vi "ClientNTTestInit.vi"(11 "Instance":u32) -> (3 "TestConfig":T1)   [LabVIEW 2019]
uses:
  ClientNTTestConfig.ctl
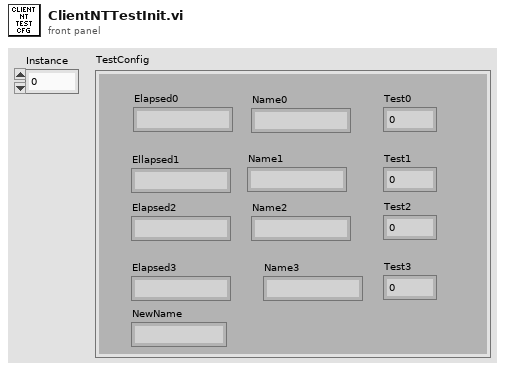
[diagram p1: front panel]
types:
  T1 = typedef "ClientNTTestConfig.ctl" = cluster{"Elapsed0":string, "Name0":string, "Test0":u32, "Ellapsed1":string, "Name1":string, "Test1":u32, "Elapsed2":string, "Name2":string, "Test2":u32, "Elapsed3":string, "Name3":string, "Test3":u32, "NewName":string}
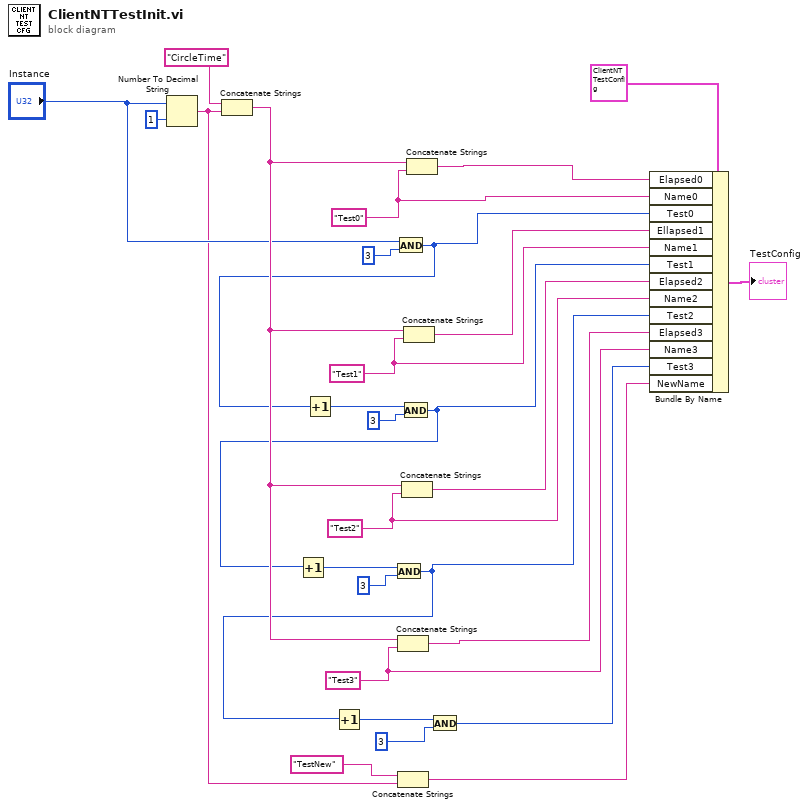
[diagram p0: block diagram]
diagram:
  w5 = "Test3" ("Name")
  w7 = "Test2" ("Name")
  w9 = "Test1" ("Name")
  w11 = "Test0" ("Name")
  n1 = Number To Decimal String(number="Instance", width (-)=i16 1) -> (decimal integer string=w3:string)
  n2 = Concatenate Strings("CircleTime" ("string"), w3) -> (w28:string)
  n3 = And(x="Instance", y=u32 3) -> (x .and. y?=w10:u32)
  n4 = Increment(x=w10) -> (x+1=w23:u32)
  n5 = Concatenate Strings(w28, w5) -> (w14:string)
  n6 = Concatenate Strings("TestNew" ("string"), w3) -> (w1:string)
  n7 = And(x=w23, y=u32 3) -> (x .and. y?=w8:u32)
  n8 = Increment(x=w8) -> (x+1=w25:u32)
  n9 = And(x=w25, y=u32 3) -> (x .and. y?=w6:u32)
  n10 = Increment(x=w6) -> (x+1=w27:u32)
  n11 = Concatenate Strings(w28, w7) -> (w13:string)
  n12 = Concatenate Strings(w28, w9) -> (w12:string)
  n13 = Concatenate Strings(w28, w11) -> (w15:string)
  n14 = And(x=w27, y=u32 3) -> (x .and. y?=w4:u32)
  n15 = Bundle By Name(cluster=T1 {"Elapsed0"="", "Name0"="", "Test0"=0, "Ellapsed1"="", "Name1"="", "Test1"=0, "Elapsed2"="", "Name2"="", "Test2"=0, "Elapsed3"="", "Name3"="", "Test3"=0, "NewName"=""} ("TestConfig"), "Elapsed0"=w15, "Name0"=w11, "Test0"=w10, "Ellapsed1"=w12, "Name1"=w9, "Test1"=w8, "Elapsed2"=w13, "Name2"=w7, "Test2"=w6, "Elapsed3"=w14, "Name3"=w5, "Test3"=w4, "NewName"=w1) -> (→"TestConfig":T1)
